vi "ImageGrabbingAveraging.vi"(6 "new":dbl[](array[numeric]), 9 "Frames grabbed":i32, 10 "Images 2D in":dbl[][](array[numeric]), 11 "y-index":i32) -> (3 "Images 2D out":dbl[][](array[numeric]))   [LabVIEW 2012, in "Image.lvclass"]
uses:
  classes/Image.lvclass
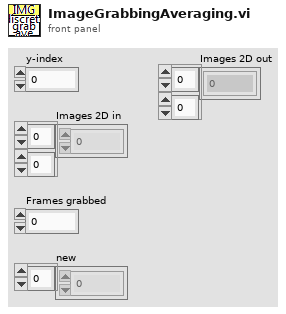
[diagram p1: front panel]
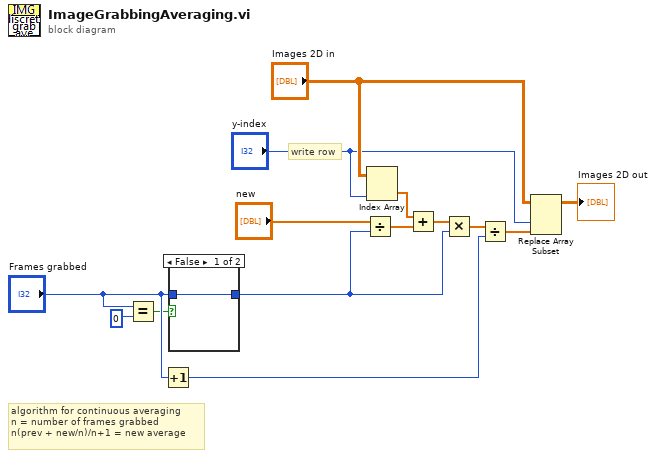
[diagram p0: block diagram]
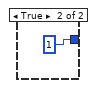
[diagram p2: hidden frame]
diagram:
  # "algorithm for continuous averaging\nn = number of frames grabbed\nn(prev + new/n)/n+1 = new average"
  # "write row"
  n1 = Equal?(x="Frames grabbed", y=0) -> (x = y?=w6:bool)
  n2 = Increment(x="Frames grabbed") -> (x+1=w5:i32)
  n3 = case shown="False" w6 {
    tunnel: "Frames grabbed" -> [w15 _]
    tunnel: [w15 1 ("Frames grabbed")] -> w11
    frame False {
    }
    frame True {
    }
  }
  n4 = Divide(x="new", y=w11) -> (x/y=w13:dbl[])
  n5 = Index Array(array="Images 2D in", index (col)="y-index") -> (element=w4:dbl[])  [unwired: 1 in]
  n6 = Add(x=w4, y=w13) -> (x+y=w10:dbl[])
  n7 = Multiply(x=w10, y=w11) -> (x*y=w12:dbl[])
  n8 = Divide(x=w12, y=w5) -> (x/y=w14:dbl[])
  n9 = Replace Array Subset(array="Images 2D in", new element=w14, index (col)="y-index") -> (→"Images 2D out":dbl[][])  [unwired: 1 in]
